vi "Post.vi"() -> ()   [LabVIEW 2020]
uses:
  <vilib>/httpClient/POSTBuffer.vi
  <vilib>/httpClient/LabVIEWHTTPClient.lvlib
panel:
  out "headers 2":string
  out "body 2":string
  in  "Data":cluster{"name":string, "job":string}={"name"="John Doe", "job"="Software Developer"}
  out "error out":errorcluster
  out "body":string
  out "headers":string
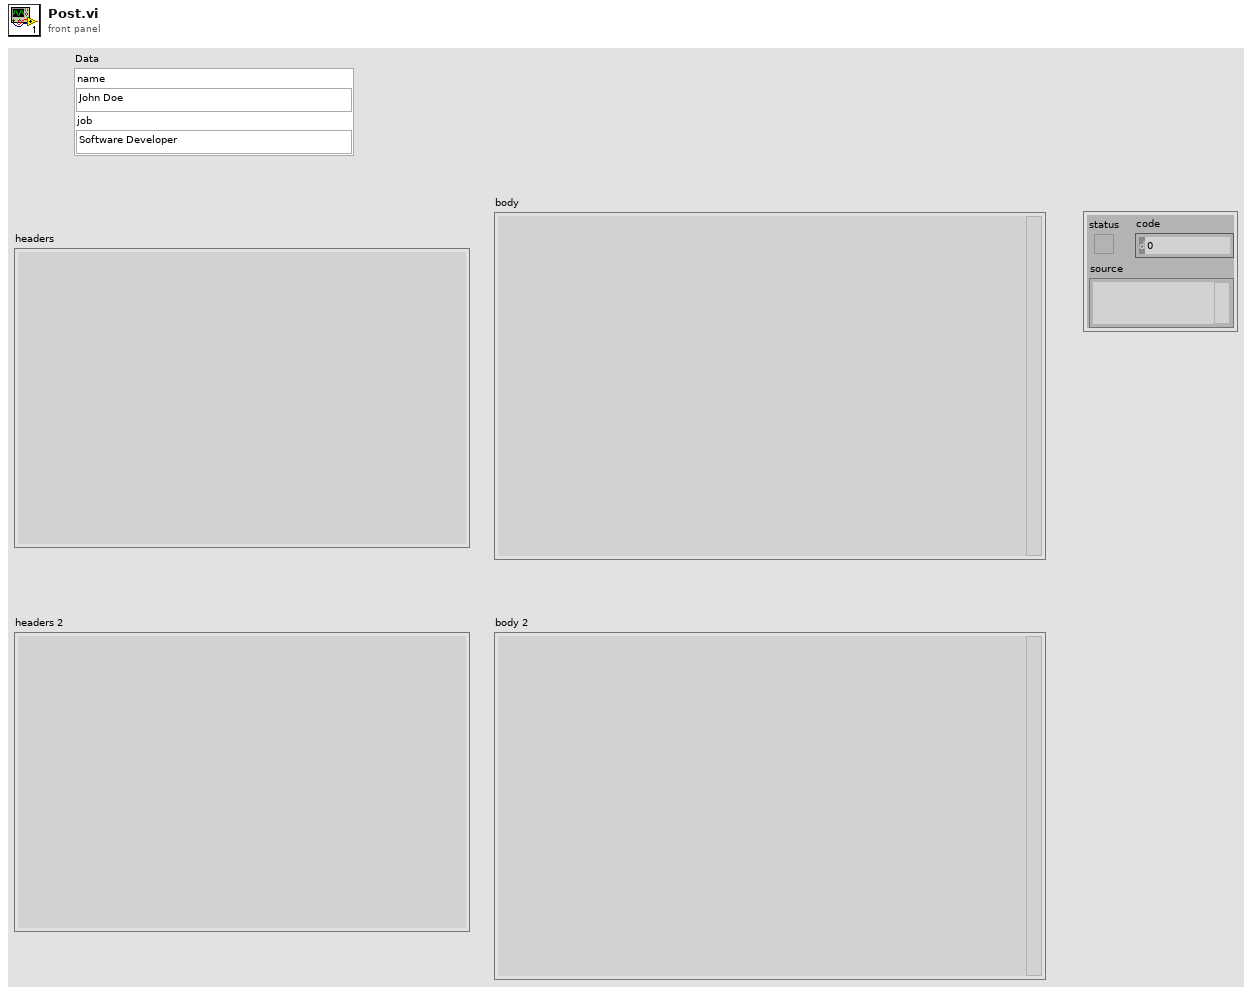
[diagram p1: front panel]
types:
  T1 = typedef "LabVIEWHTTPClient.lvlib/ClientHandle.ctl" = refnum<k1>
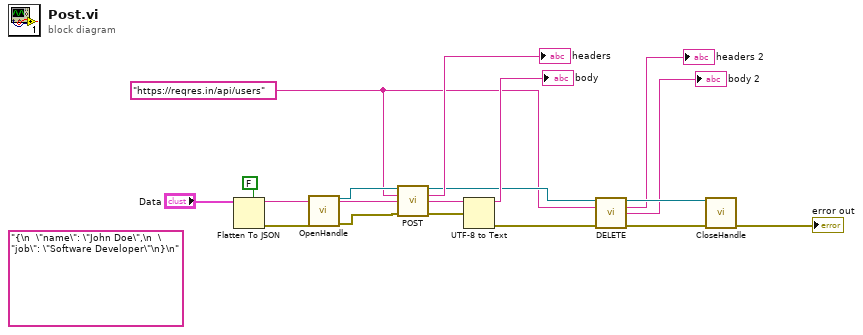
[diagram p0: block diagram]
diagram:
  (unwired) "{\n  \"name\": \"John Doe\",\n  \"job\": \"Software Developer\"\n}\n" ("buffer")
  w3 = "https://reqres.in/api/users" ("url")
  n1 = Flatten To JSON(enable LabVIEW extensions? (T)=FALSE, anything="Data") -> (JSON string=w16:string, 11:w10:errorcluster)  [unwired: 1 in]
  n2 = call <vilib>:"OpenHandle.vi"("error in (no error)"=w10) -> ("client handle out"=w11:T1, "error out"=w9:errorcluster)  [unwired: 13 in]
  n3 = call-poly <vilib>:"POST.vi"("client handle"=w11, "url"=w3, "buffer"=w16, "error in (no error)"=w9) -> ("client handle out"=w7:T1, "headers"=→"headers":string, "body"=w14:string, "error out"=w12:errorcluster)  [unwired: 8 in]
  n4 = UTF-8 to Text(8:w12, 11:w14) -> (0:w8:errorcluster, 3:→"body":string)  [unwired: 1 in]
  n5 = call <vilib>:"DELETE.vi"("client handle"=w7, "url"=w3, "error in (no error)"=w8) -> ("client handle out"=w4:T1, "headers"=→"headers 2":string, "body"=→"body 2":string, "error out"=w6:errorcluster)  [unwired: 9 in]
  n6 = call <vilib>:"CloseHandle.vi"("client handle"=w4, "error in (no error)"=w6) -> ("error out"=→"error out":errorcluster)  [unwired: 13 in]
